vi "Image to luminosity gradient complex map.vi"(2 "Error In":errorcluster, 3 "ROI to crop (pixels)":T1={"Xmax"=2147483647, "Ymax"=2147483647, "Xmin"=0, "Ymin"=0}, 4 "Image":T2) -> (0 "Error Out":errorcluster, 1 "Luminosity gradient map (complex)":cdb[][](array[numeric]))   [LabVIEW 2014]
uses:
  <vilib>/vision/Image Controls.llb/IMAQ Image.ctl
  Typedefs/ROI bounds.ctl
  <vilib>/Analysis/2dsp.llb/2D Convolution (DBL).vi
  <vilib>/vision/NI_Vision_Development_Module.lvlib
  <vilib>/Analysis/NI_AALPro.lvlib
panel:
  # "Paul Nathan 03/06/2015, 18/06/2015"
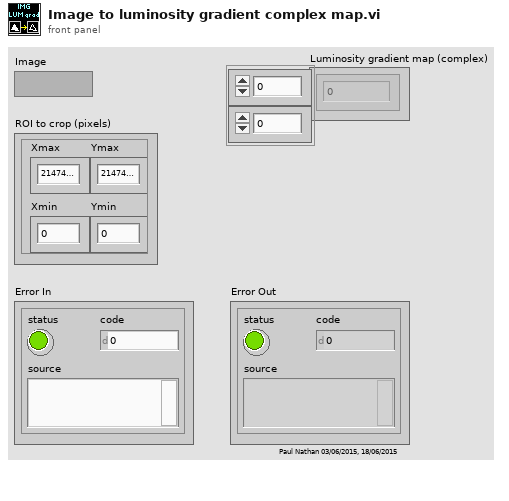
[diagram p1: front panel]
types:
  T1 = typedef "ROI bounds.ctl" = cluster{"Xmax":i32, "Ymax":i32, "Xmin":i32, "Ymin":i32}
  T2 = typedef "IMAQ Image.ctl" = refnum<image>
  T3 = cluster{"Red (or Hue) value":u8, "Green (or Sat) value":u8, "Blue (or Light or Val) value":u8}[][]
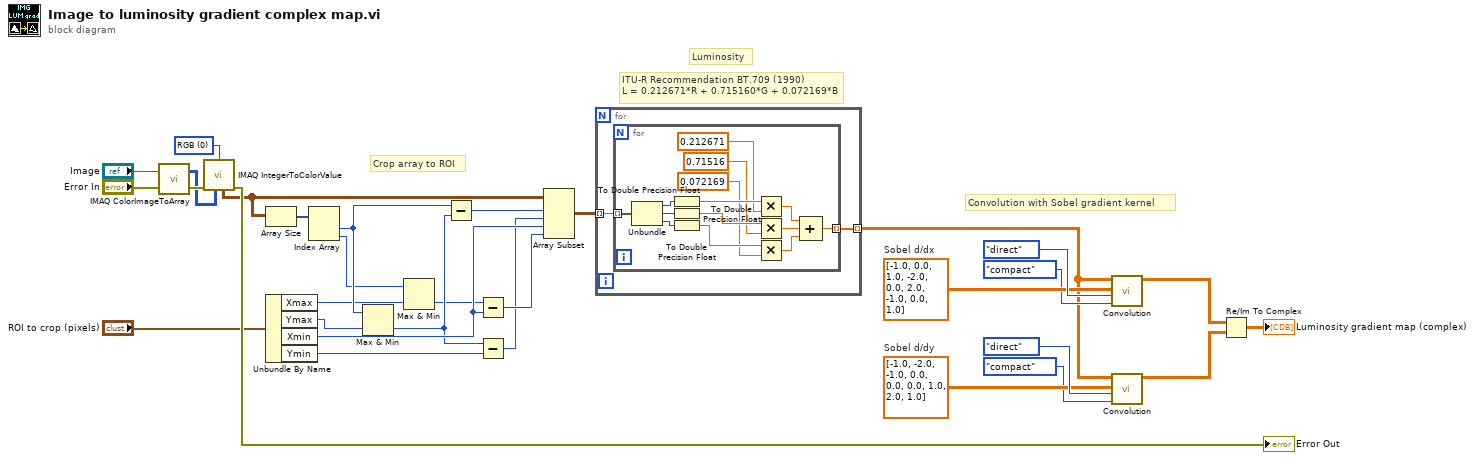
[diagram p0: block diagram]
diagram:
  w24 = dbl[][] [[-1.0, -2.0, -1.0], [0.0, 0.0, 0.0], [1.0, 2.0, 1.0]]  # Sobel d/dy
  w27 = dbl[][] [[-1.0, 0.0, 1.0], [-2.0, 0.0, 2.0], [-1.0, 0.0, 1.0]]  # Sobel d/dx
  w29 = u16 0 items=["RGB", "HSL", "HSV", "HSI"] ("Color Mode")
  # "Crop array to ROI"
  # "Convolution with Sobel gradient kernel"
  # "Luminosity"
  # "ITU-R Recommendation BT.709 (1990)\nL = 0.212671*R + 0.715160*G + 0.072169*B"
  n1 = call "IMAQ ColorImageToArray"("Image"="Image", "error in (no error)"="Error In") -> ("Image Pixels (U32)"=w30:u32[][], "error out"=w31:errorcluster)  [unwired: 2 in, 1 out]
  n2 = call "IMAQ IntegerToColorValue"("error in (no error)"=w31, "2D U32 array"=w30, "Color Mode"=w29) -> ("2D Color value array"=w12:T3, "error out"=→"Error Out":errorcluster)  [unwired: 2 in, 2 out]
  n3 = Array Size(array=w12) -> (size(s)=w15:i32[])
  n4 = Unbundle By Name("ROI to crop (pixels)") -> ("Xmax"=w3:i32, "Ymax"=w7:i32, "Xmin"=w10:i32, "Ymin"=w14:i32)
  n5 = Index Array(array=w15) -> (element #1=w6:i32, element #2=w2:i32)  [unwired: 2 in]
  n6 = Max & Min(x=w6, y=w7) -> (min(x,y)=w5:i32)  [unwired: 1 out]
  n7 = Max & Min(x=w2, y=w3) -> (min(x,y)=w1:i32)  [unwired: 1 out]
  n8 = Subtract(x=w6, y=w5) -> (x-y=w8:i32)
  n9 = Subtract(x=w1, y=w10) -> (x-y=w9:i32)
  n10 = Subtract(x=w5, y=w14) -> (x-y=w4:i32)
  n11 = Array Subset(array=w12, index (row)=w8, length (row)=w4, index (col)=w10, length (col)=w9) -> (w11:T3)
  n12 = for {
    tunnel: w11 -> [w33] mode=indexing
    tunnel: [w32] -> w13 mode=indexing
    n13 = for {
      tunnel: w33 -> [w47] mode=indexing
      tunnel: [w34] -> w32 mode=indexing
      n14 = Unbundle(w47) -> ("Red (or Hue) value"=w46:u8, "Green (or Sat) value"=w44:u8, "Blue (or Light or Val) value"=w45:u8)
      n15 = To Double Precision Float(number=w46) -> (double precision float=w43:dbl)
      n16 = To Double Precision Float(number=w44) -> (double precision float=w42:dbl)
      n17 = To Double Precision Float(number=w45) -> (double precision float=w41:dbl)
      n18 = Multiply(x=w43, y=0.212671) -> (x*y=w37:dbl)
      n19 = Multiply(x=w42, y=0.71516) -> (x*y=w36:dbl)
      n20 = Multiply(x=w41, y=0.072169) -> (x*y=w35:dbl)
      n21 = Compound Arithmetic op=ADD(w37, w36, w35) -> (w34:dbl)
    }
  }
  n22 = call-poly <vilib>:"Convolution.vi"("output size"=enum32{"full", "size X", "compact"}."compact", "algorithm"=enum32{"direct", "frequency domain"}."direct", "Y"=w27, "X"=w13) -> ("X * Y"=w23:dbl[][])  [unwired: 6 in, 1 out]
  n23 = call-poly <vilib>:"Convolution.vi"("output size"=enum32{"full", "size X", "compact"}."compact", "algorithm"=enum32{"direct", "frequency domain"}."direct", "Y"=w24, "X"=w13) -> ("X * Y"=w22:dbl[][])  [unwired: 6 in, 1 out]
  n24 = Re/Im To Complex(1:w22, 2:w23) -> (0:→"Luminosity gradient map (complex)":cdb[][])
